vi "IT8800-Configure Resource.vi"(8 "error in (no error)":errorcluster, 11 "ITech Setting In in":T1 {"Stop Bits" items=["1.0"=10, "2.0"=20]; "Baud Rate" items=["2400"=2400, "4800"=4800, "9600"=9600, "19200"=19200]}) -> (0 "error out":errorcluster, 3 "ITech Setting In out":T1 {"Stop Bits" items=["1.0"=10, "2.0"=20]; "Baud Rate" items=["2400"=2400, "4800"=4800, "9600"=9600, "19200"=19200]})   [LabVIEW 2018]
uses:
  Data Def/IT8800-Setting.ctl
  <vilib>/Instr/_visa.llb/VISA Configure Serial Port (Instr).vi
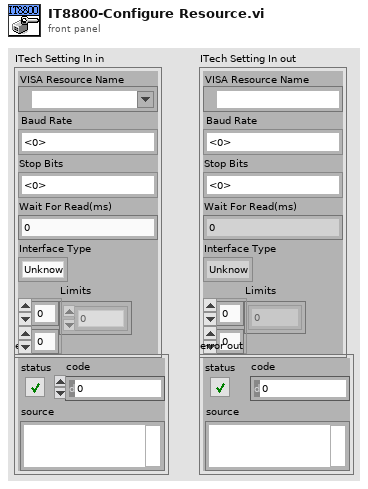
[diagram p1: front panel]
types:
  T1 = typedef "IT8800-Setting.ctl" = cluster{"VISA Resource Name":refnum<visa-resource-name>, "Baud Rate":u32, "Stop Bits":u16, "Wait For Read(ms)":u32, "Interface Type":enum16{"Unknow", "GPIB", "VXI", "GPIB-VXI", "Serial", "PXI", "TCPIP", "USB", "FireWire"}, "Limits":dbl[][]}
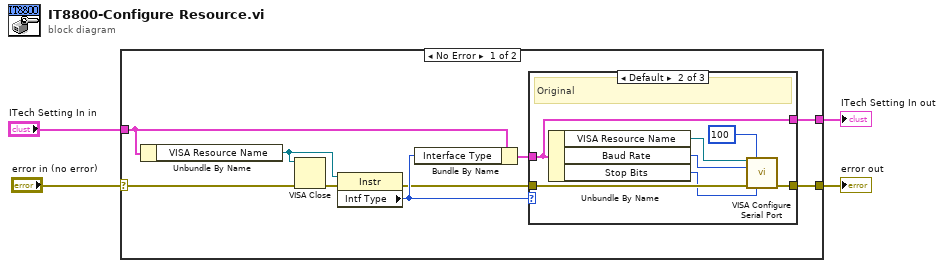
[diagram p0: block diagram]
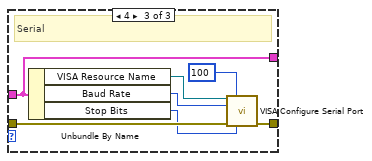
[diagram p3: hidden frame]
diagram:
  n1 = case shown="No Error" "error in (no error)" {
    selector: "error in (no error)" -> [w5 w30]
    tunnel: [w11 w31] -> w4
    tunnel: "ITech Setting In in" -> [w9 w31]
    tunnel: [w8 w30] -> w2
    frame No Error {
      n2 = Unbundle By Name(w9) -> ("VISA Resource Name"=w6:refnum<visa-resource-name>)
      n3 = VISA Close(VISA resource name=w6, error in (no error)=w5) -> (error out=w13:errorcluster)
      n4 = property class="Instr"(reference=w6, error in=w13) -> (error out=w7:errorcluster, "Intf Type"=w12:u16)  [unwired: 1 out]
      n5 = Bundle By Name(cluster=w9, "Interface Type"=w12) -> (w10:T1)
      n6 = case shown="Default" w12 {
        tunnel: w7 -> [w15 w21 w28]
        tunnel: [w15 w20 w27] -> w8
        tunnel: w10 -> [w14 w17 w24]
        tunnel: [w14 w17 w24] -> w11
        frame 7 {
          # "USB"
        }
        frame Default {
          # "Original"
          n7 = Unbundle By Name(w17) -> ("VISA Resource Name"=w16:refnum<visa-resource-name>, "Baud Rate"=w19:u32, "Stop Bits"=w18:u16)
          n8 = call-poly "VISA Configure Serial Port"("VISA resource name"=w16, "timeout (10sec)"=u32 100, "baud rate (9600)"=w19, "error in (no error)"=w21, "stop bits (10: 1 bit)"=w18) -> ("error out"=w20:errorcluster)  [unwired: 9 in, 1 out]
        }
        frame 4 {
          # "Serial"
          n9 = Unbundle By Name(w24) -> ("VISA Resource Name"=w23:refnum<visa-resource-name>, "Baud Rate"=w26:u32, "Stop Bits"=w25:u16)
          n10 = call-poly "VISA Configure Serial Port"("VISA resource name"=w23, "timeout (10sec)"=u32 100, "baud rate (9600)"=w26, "error in (no error)"=w28, "stop bits (10: 1 bit)"=w25) -> ("error out"=w27:errorcluster)  [unwired: 9 in, 1 out]
        }
      }
    }
    frame Error {
    }
  }
  "ITech Setting In out" <- w4
  "error out" <- w2
